vi "SavePythonFile.vi"(9 "path":path, 11 "Code":string) -> ()   [LabVIEW 2020]
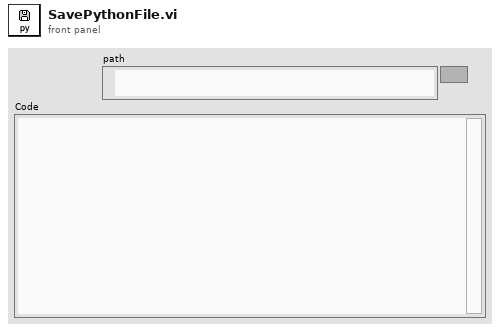
[diagram p1: front panel]
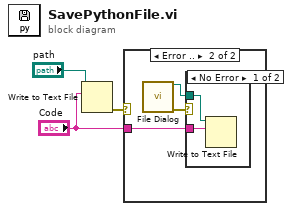
[diagram p0: block diagram]
diagram:
  n1 = Write to Text File(file (use dialog)="path", text="Code") -> (error out=w2:errorcluster)  [unwired: 2 in, 2 out]
  n2 = case shown="Error .." w2 {
    tunnel: "Code" -> [_ w5]
    frame No Error {
    }
    frame Error {
      n3 = call "File Dialog"() -> ("selected path"=w4:path, "error out"=w6:errorcluster)  [unwired: 12 in, 2 out]
      n4 = case shown="No Error" w6 {
        tunnel: w5 -> [w8 _]
        tunnel: w4 -> [w7 _]
        frame No Error {
          n5 = Write to Text File(file (use dialog)=w7, text=w8) -> ()  [unwired: 2 in, 3 out]
        }
        frame Error {
        }
      }
    }
  }
